vi "TestLicor.vi"() -> ()   [LabVIEW 2010]
uses:
  <vilib>/Instr/_visa.llb/VISA Configure Serial Port (Instr).vi
panel:
  in  "flow control (0:none)":u16(ring) caption="Ablaufsteuerung (0: keine)" items=["Keine", "XON/XOFF", "RTS/CTS", "XON/XOFF & RTS/CTS", "DTR/DSR", "XON/XOFF & DTR/DSR"]
  in  "Stopp":bool
  out "vomLicor":string
  in  "Schreibpuffer":string
  in  "senden":bool
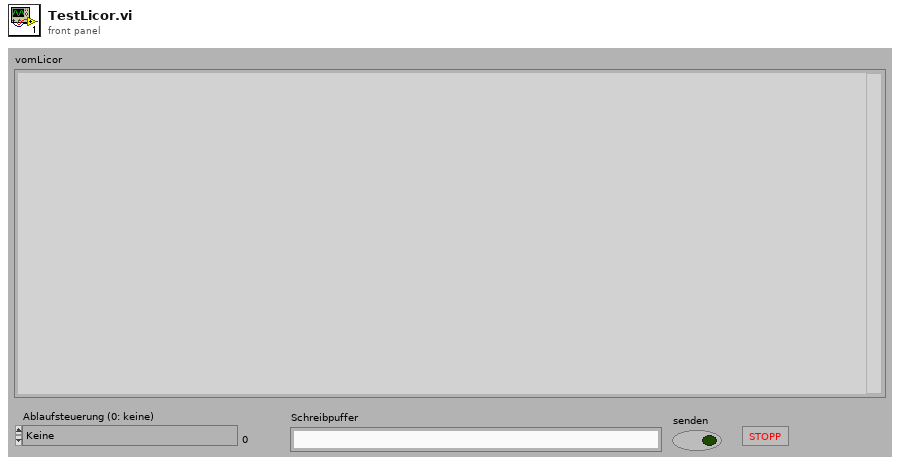
[diagram p1: front panel]
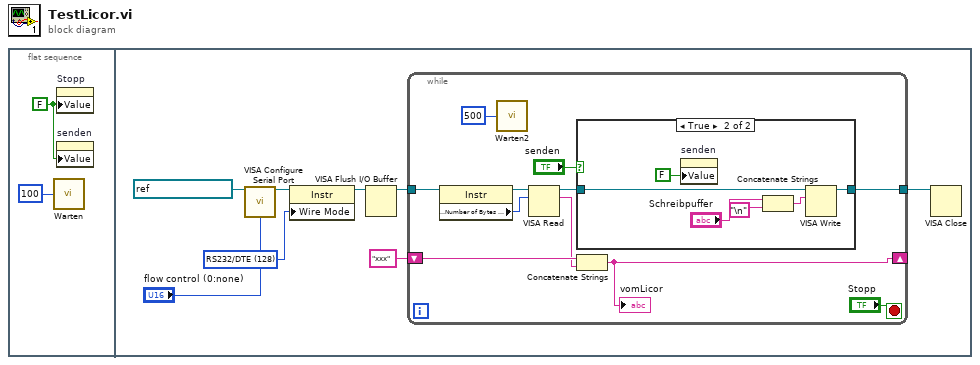
[diagram p0: block diagram]
diagram:
  n1 = flat-sequence {
    frame #0 {
      w1 = FALSE ("Stopp")
      n2 = call "Warten"("Count(mSec)"=u32 100) -> ()  [unwired: 1 out]
      n3 = property on="Stopp" class="Bool. (strikt)"("Value"=w1) -> ()  [unwired: 2 in, 2 out]
      n4 = property on="senden" class="Bool. (strikt)"("Value"=w1) -> ()  [unwired: 2 in, 2 out]
    }
    frame #1 {
      w7 = i16 128 items=["Unknown"=-1, "RS485/Wire4"=0, "RS485/Wire2-EchoDTR"=1, "RS485/Wire2-CtrlDTR"=2, "RS485/Wire2-Auto"=3, "RS232/DTE"=128, "RS232/DCE"=129, "RS232/AUTO"=130] ("Serial Settings:Wire Mode")
      n5 = call-poly "VISA Configure Serial Port"("VISA resource name"=refnum<visa-resource-name> "ASRL1::INSTR", "flow control (0:none)"="flow control (0:none)") -> ("VISA resource name out"=w4:refnum<visa-resource-name>)  [unwired: 12 in, 1 out]
      n6 = property class="Instr"(reference=w4, "Wire Mode"=w7) -> (reference out=w6:refnum<visa-resource-name>)  [unwired: 1 in, 1 out]
      n7 = VISA Flush I/O Buffer(VISA resource name=w6) -> (VISA resource name out=w5:refnum<visa-resource-name>)  [unwired: 2 in, 1 out]
      n8 = while {
        tunnel: w5 -> [w17]
        shift-right: [w19] -> _
        shift-left: "xxx" -> [w21]
        tunnel: [w13] -> w9
        stop <- "Stopp" stop-if-true
        n9 = property class="Instr"(reference=w17) -> (reference out=w16:refnum<visa-resource-name>, "Serial Settings:Number of Bytes at Serial Port"=w15:u32)  [unwired: 1 in, 1 out]
        n10 = call "Warten2"("Count(mSec)"=u32 500) -> ()  [unwired: 1 out]
        n11 = VISA Read(VISA resource name=w16, byte count=w15) -> (VISA resource name out=w14:refnum<visa-resource-name>, read buffer=w20:string)  [unwired: 1 in, 2 out]
        n12 = case shown="True" "senden" {
          tunnel: w14 -> [w22 w25]
          tunnel: [w22 w24] -> w13
          frame False {
          }
          frame True {
            n13 = property on="senden" class="Bool. (strikt)"("Value"=FALSE ("senden")) -> ()  [unwired: 2 in, 2 out]
            n14 = Concatenate Strings("Schreibpuffer", "\n") -> (w26:string)
            n15 = VISA Write(VISA resource name=w25, write buffer=w26) -> (VISA resource name out=w24:refnum<visa-resource-name>)  [unwired: 1 in, 2 out]
          }
        }
        n16 = Concatenate Strings(w21, w20) -> (w19:string)
        "vomLicor" <- w19
      }
      n17 = VISA Close(VISA resource name=w9) -> ()  [unwired: 1 in, 1 out]
    }
  }
